vi "Stop.vi"(0 "Universal Robot.lvclass in":refnum<class "Universal Robot.lvclass">, 5 "error in (no error)":errorcluster) -> (14 "Universal Robot.lvclass out":refnum<class "Universal Robot.lvclass">, 19 "error out":errorcluster)   [LabVIEW 2016, in "Universal Robot.lvclass"]
uses:
  Universal Robot.lvclass
  Universal Robot.lvclass/Universal Robot.ctl
  DashboardServer/Dashboard Server.lvclass
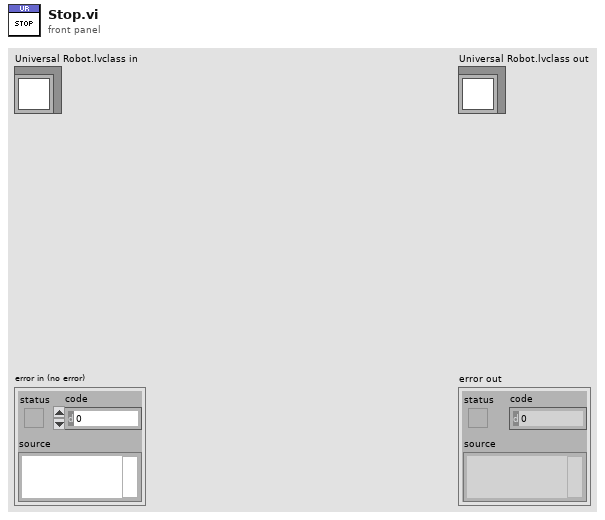
[diagram p1: front panel]
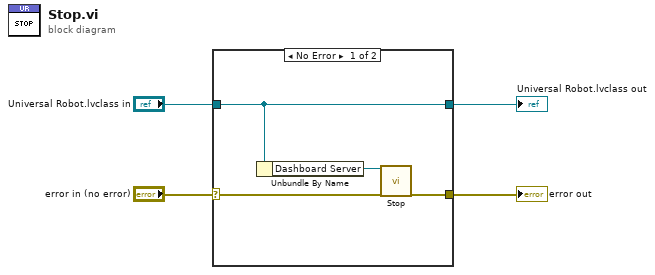
[diagram p0: block diagram]
diagram:
  n1 = case shown="No Error" "error in (no error)" {
    selector: "error in (no error)" -> [w5 w10]
    tunnel: [w7 w10] -> w3
    tunnel: "Universal Robot.lvclass in" -> [w8 w9]
    tunnel: [w8 w9] -> w1
    frame No Error {
      n2 = Unbundle By Name(w8) -> ("Dashboard Server"=w6:refnum<class "Dashboard Server.lvclass">)
      n3 = call-dynamic "Stop.vi"("DashboardServer in"=w6, "error in (no error)"=w5) -> ("error out"=w7:errorcluster)  [unwired: 16 in, 1 out]
    }
    frame Error {
    }
  }
  "error out" <- w3
  "Universal Robot.lvclass out" <- w1
